vi "JSONRPC-ReadablesWritablesToString.vi"(11 "readables/writables":T1(array[cluster])) -> (3 "Output":string)   [LabVIEW 2020]
uses:
  JSONRPC-ArrayToString_String.vi
panel:
  # "ReadablesWritablesToString"
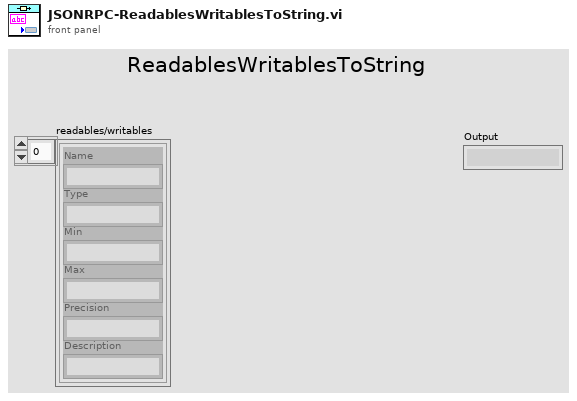
[diagram p1: front panel]
types:
  T1 = cluster{"Name":string, "Type":string, "Min":string, "Max":string, "Precision":string, "Description":string}[]
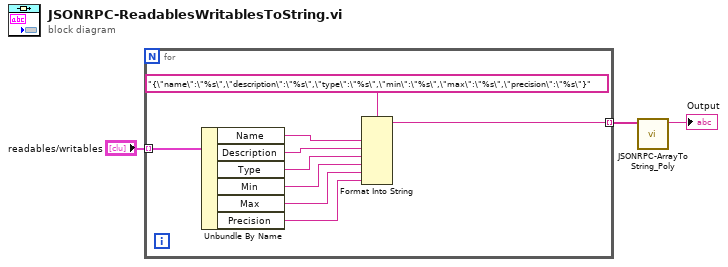
[diagram p0: block diagram]
diagram:
  n1 = for {
    tunnel: "readables/writables" -> [w12] mode=indexing
    tunnel: [w9] -> w3 mode=indexing
    n2 = Unbundle By Name(w12) -> ("Name"=w10:string, "Description"=w8:string, "Type"=w7:string, "Min"=w6:string, "Max"=w5:string, "Precision"=w4:string)
    n3 = Format Into String(format string="{\"name\":\"%s\",\"description\":\"%s\",\"type\":\"%s\",\"min\":\"%s\",\"max\":\"%s\",\"precision\":\"%s\"}", w10, w8, w7, w6, w5, w4) -> (resulting string=w9:string)  [unwired: 2 in, 1 out]
  }
  n4 = call-poly "JSONRPC-ArrayToString_Poly.vi"("Array"=w3) -> ("Output"=→"Output":string)  [unwired: 10 in]
